vi "ScopeInfoToString(Array).vi"(10 "info":T1={"Name"="", "N"=-4.9992e-05, "t0"=1e-08, "dt"=0.0, "offset"=1.0, "gain"=0.0, "coupling"="50 ohms", "impedance"="", "range"=0.0}, 11 "precision (12)":i16=12) -> (1 "Headder Array":string[](array[string]), 2 "Element Names":string[](array[string]), 3 "info string array":string[](array[string])=["10000.000000000000", "-0.000049992000", "0.000000010000", "0.000000000000", "1.000000000000", "DC", "50 ohms", "4.000000000000"])   [LabVIEW 2011]
uses:
  scopeTraceInfo_TypDEf.ctl
panel:
  out "x-y":u32
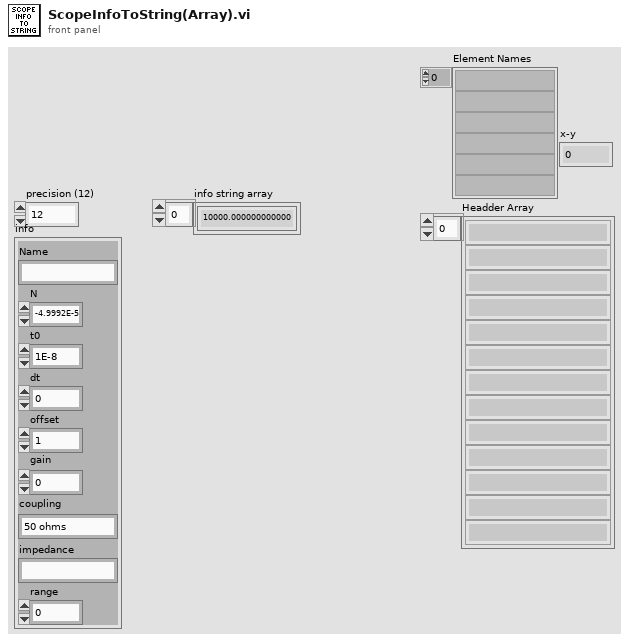
[diagram p1: front panel]
types:
  T1 = typedef "scopeTraceInfo_TypDEf.ctl" = cluster{"Name":string, "N":dbl, "t0":dbl, "dt":dbl, "offset":dbl, "gain":dbl, "coupling":string, "impedance":string, "range":dbl}
  T2 = typedef "Type Descriptor Enumeration__ogtk.ctl" = enum8{"<Null>", "I8", "I16", "I32", "I64", "U8", "U16", "U32", "U64", "SGL", "DBL", "EXT", "CSG", "CDB", "CXT", "0x0F", "0x10", "0x11", "0x12", "0x13", "0x14", "Enum U8", "Enum U16", "Enum U32", "Enum U64", "SGL PQ", "DBL PQ", "EXT PQ", "CSG PQ", "CDB PQ", "CXT PQ", "0x1F", "0x20", "Boolean", "0x22", "0x23", "0x24", "0x25", "0x26", "0x27", "0x28", "0x29", "0x2A", "0x2B", "0x2C", "0x2D", "0x2E", "0x2F", "String", "0x31", "Path", "Pict", "0x34", "0x35", "0x36", "DAQ", "0x38", "0x39", "0x3A", "0x3B", "0x3C", "0x3D", "0x3E", "0x3F", "Array", "0x41", "0x42", "0x43", "0x44", "0x45", "0x46", "0x47", "0x48", "0x49", "0x4A", "0x4B", "0x4C", "0x4D", "0x4E", "0x4F", "Cluster", "0x51", "0x52", "Variant", "Waveform", "0x55", "0x56", "0x57", "0x58", "0x59", "0x5A", "0x5B", "0x5C", "0x5D", "0x5E", "0x5F", "0x60", "0x61", "0x62", "0x63", "0x64", "0x65", "0x66", "0x67", "0x68", "0x69", "0x6A", "0x6B", "0x6C", "0x6D", "0x6E", "0x6F", "Refnum"}
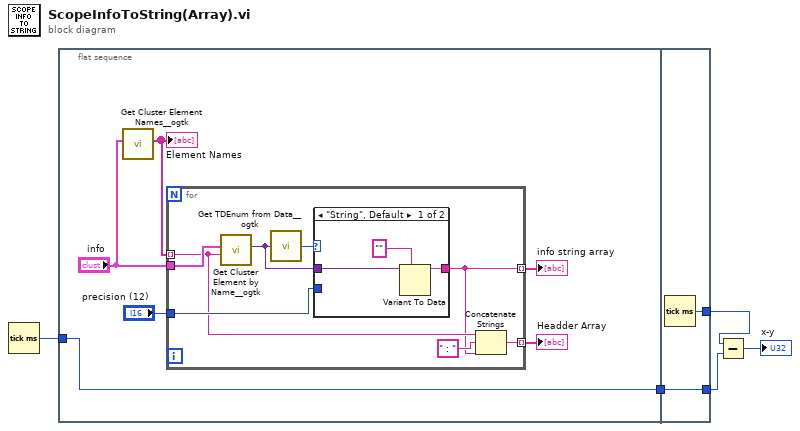
[diagram p0: block diagram]
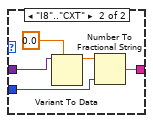
[diagram p2: hidden frame]
diagram:
  n1 = Tick Count (ms)() -> (millisecond timer value=w5:u32)
  n2 = flat-sequence {
    tunnel: w5 -> [w6]
    tunnel: [w6] -> w2
    tunnel: [w29] -> w4
    tunnel: w2 -> [w29]
    tunnel: [w28] -> w1
    frame #0 {
      n3 = call "Get Cluster Element Names__ogtk.vi"("Cluster"="info") -> ("Element Names"=w9:string[])  [unwired: 9 in, 1 out]
      "Element Names" <- w9
      n4 = for {
        tunnel: "info" -> [w19]
        tunnel: w9 -> [w15] mode=indexing
        tunnel: [w13] -> w11 mode=indexing
        tunnel: "precision (12)" -> [w16]
        tunnel: [w12] -> w7 mode=indexing
        n5 = call "Get Cluster Element by Name__ogtk.vi"("Element Name"=w15, "Cluster"=w19) -> ("VElement"=w17:variant)  [unwired: 7 in, 2 out]
        n6 = call "Get TDEnum from Data__ogtk.vi"("Data"=w17) -> ("Type Descriptor Enumeration"=w18:T2)  [unwired: 4 in]
        n7 = case shown="\"String\", Default" w18 {
          tunnel: w17 -> [w21 w27]
          tunnel: [w20 w24] -> w13
          tunnel: w16 -> [_ w23]
          frame "String", Default {
            n8 = Variant To Data(type="", Variant=w21) -> (data=w20:string)  [unwired: 1 in, 1 out]
          }
          frame "I8".."CXT" {
            n9 = Variant To Data(type=0.0, Variant=w27) -> (data=w25:dbl)  [unwired: 1 in, 1 out]
            n10 = Number To Fractional String(number=w25, precision (6)=w23) -> (F-format string=w24:string)  [unwired: 2 in]
          }
        }
        n11 = Concatenate Strings(w15, " : " ("string"), w13) -> (w12:string)
      }
      "info string array" <- w11
      "Headder Array" <- w7
    }
    frame #1 {
      n12 = Tick Count (ms)() -> (millisecond timer value=w28:u32)
    }
  }
  n13 = Subtract(x=w1, y=w4) -> (x-y=→"x-y":u32)
